vi "soundGlobal.vi"() -> ()   [LabVIEW 2010]
panel:
  out "ON":bool
  in  "stop":bool
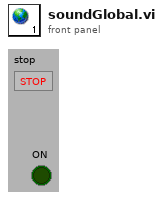
[diagram p1: front panel]
diagram:
